vi "FILO string equal.vi"(0 "Array":string[](array[string]), 2 "Array size":i32, 7 "String":string) -> (4 "Array out":string[](array[string]))   [LabVIEW 2014]
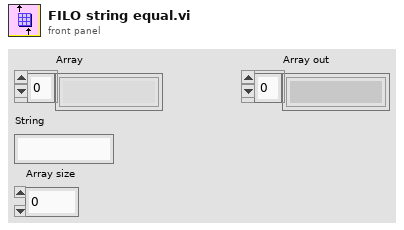
[diagram p1: front panel]
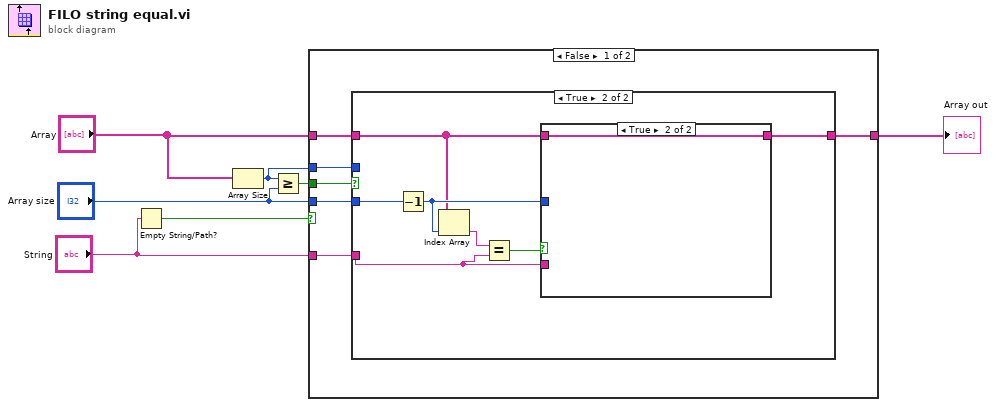
[diagram p0: block diagram]
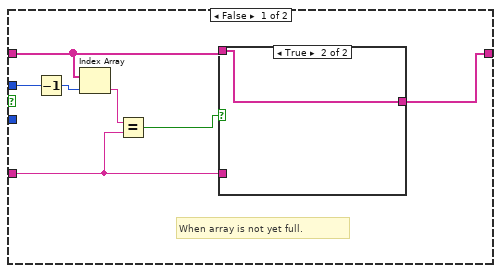
[diagram p2: hidden frame]
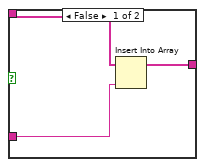
[diagram p3: hidden frame]
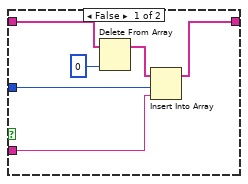
[diagram p4: hidden frame]
diagram:
  n1 = Empty String/Path?(string/path="String") -> (empty?=w7:bool)
  n2 = Array Size(array="Array") -> (size(s)=w1:i32)
  n3 = Greater Or Equal?(x=w1, y="Array size") -> (x >= y?=w6:bool)
  n4 = case shown="False" w7 {
    tunnel: w6 -> [w13 _]
    tunnel: "Array" -> [w12 w39]
    tunnel: "String" -> [w11 _]
    tunnel: [w10 w39] -> w2
    tunnel: "Array size" -> [w9 _]
    tunnel: w1 -> [w8 _]
    frame False {
      n5 = case shown="True" w13 {
        tunnel: [w20 w31] -> w10
        tunnel: w12 -> [w17 w28]
        tunnel: w11 -> [w16 w26]
        tunnel: w9 -> [_ w30]
        tunnel: w8 -> [w19 _]
        frame False {
          # "When array is not yet full."
          n6 = Decrement(x=w19) -> (x-1=w18:i32)
          n7 = Index Array(array=w17, index=w18) -> (element=w15:string)
          n8 = Equal?(x=w15, y=w16) -> (x = y?=w14:bool)
          n9 = case shown="True" w14 {
            tunnel: [w23 w24] -> w20
            tunnel: w17 -> [w22 w24]
            tunnel: w16 -> [w21 _]
            frame False {
              n10 = Insert Into Array(array=w22, new element=w21) -> (w23:string[])  [unwired: 1 in]
            }
            frame True {
            }
          }
        }
        frame True {
          n11 = Decrement(x=w30) -> (x-1=w29:i32)
          n12 = Index Array(array=w28, index=w29) -> (element=w27:string)
          n13 = Equal?(x=w27, y=w26) -> (x = y?=w25:bool)
          n14 = case shown="True" w25 {
            tunnel: [w35 w38] -> w31
            tunnel: w29 -> [w34 _]
            tunnel: w28 -> [w33 w38]
            tunnel: w26 -> [w32 _]
            frame False {
              n15 = Delete From Array(array=w33, index=0) -> (array with subset deleted=w36:string[])  [unwired: 1 in, 1 out]
              n16 = Insert Into Array(array=w36, index=w34, new element=w32) -> (w35:string[])
            }
            frame True {
            }
          }
        }
      }
    }
    frame True {
      # "String is empty."
    }
  }
  "Array out" <- w2
